vi "RefereeVSS.vi"(6 "RX":bool, 10 "element":u8[](array[numeric]), 11 "VSS_Ref 4":T1={"FoulQuadrantVSS"=enum."NO_QUADRANT", "TeamColorVSS"=enum."YELLOW", "HalfVSS"=enum."NO_HALF", "Foul"=enum."FREE_KICK", "timestamp"=0.0}) -> (0 "error out 2":errorcluster, 1 "VSS_Ref 3":T1={"FoulQuadrantVSS"=enum."NO_QUADRANT", "TeamColorVSS"=enum."YELLOW", "HalfVSS"=enum."NO_HALF", "Foul"=enum."FREE_KICK", "timestamp"=0.0})   [LabVIEW 2023]
uses:
  Referee_class/Referee.lvclass
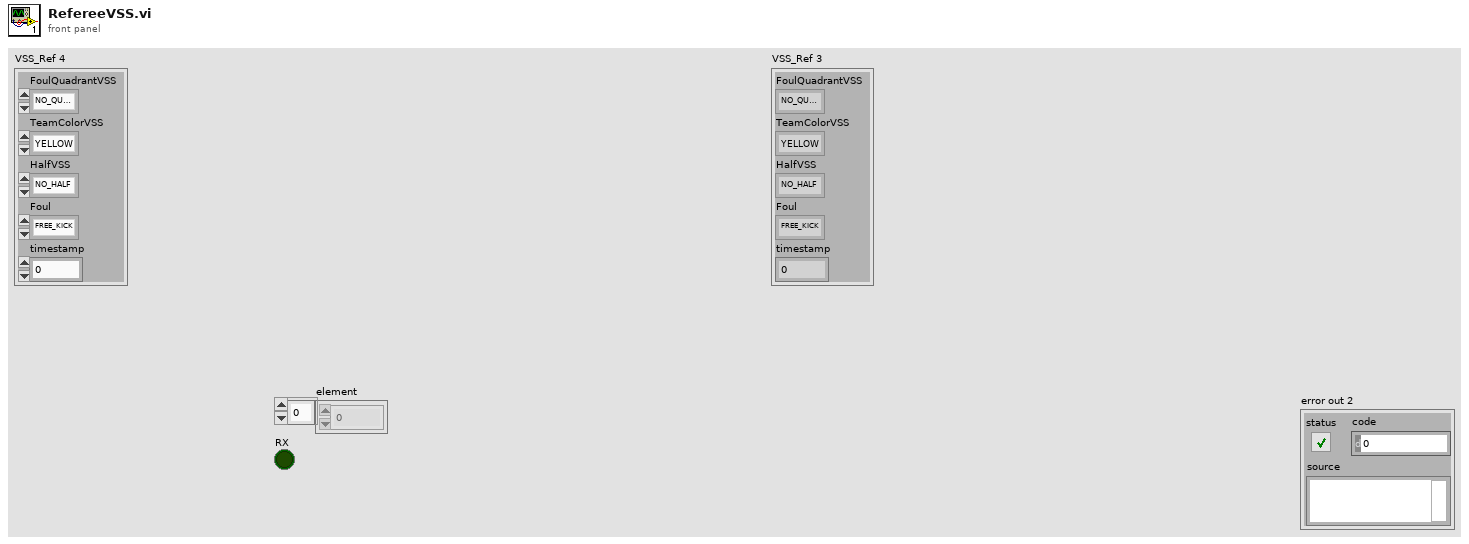
[diagram p1: front panel]
types:
  T1 = typedef "VSS_Ref.ctl" = cluster{"FoulQuadrantVSS":enum16{"NO_QUADRANT", "QUADRANT_1", "QUADRANT_2", "QUADRANT_3", "QUADRANT_4"}, "TeamColorVSS":enum16{"BLUE", "YELLOW", "NONE"}, "HalfVSS":enum16{"NO_HALF", "FIRST_HALF", "SECOND_HALF", "OVERTIME_FIRST_HALF", "OVERTIME_SECOND_HALF", "PENALTY_SHOOTOUS"}, "Foul":enum16{"FREE_KICK", "PENALTY_KICK", "GOAL_KICK", "FREE_BALL", "KICKOFF", "STOP", "GAME_ON", "HALT"}, "timestamp":dbl}
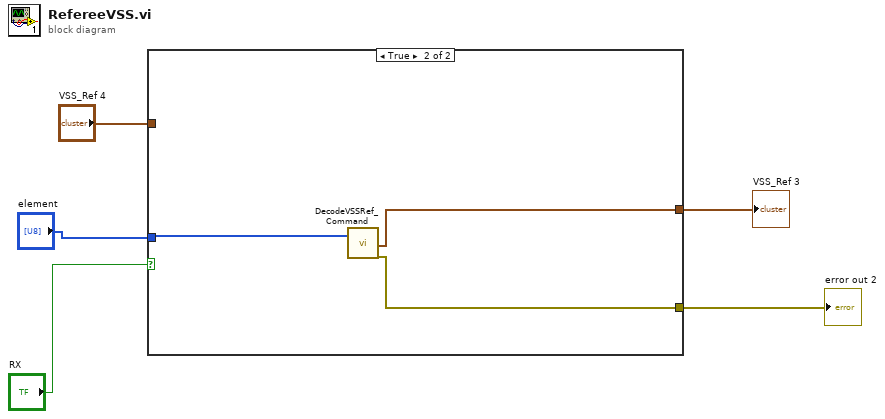
[diagram p0: block diagram]
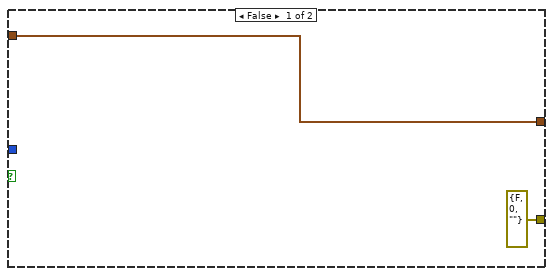
[diagram p2: hidden frame]
diagram:
  n1 = case shown="True" "RX" {
    tunnel: "element" -> [_ w10]
    tunnel: [errorcluster {"status"=FALSE, "code"=0, "source"=""} ("error out") w9] -> w3
    tunnel: [w6 w8] -> w2
    tunnel: "VSS_Ref 4" -> [w6 _]
    frame False {
    }
    frame True {
      n2 = call "DecodeVSSRef_Command.vi"("element"=w10) -> ("VSS_Ref 3"=w8:T1, "error out"=w9:errorcluster)  [unwired: 17 in]
    }
  }
  "error out 2" <- w3
  "VSS_Ref 3" <- w2
